vi "test Acyclic Loopback with SDI.vi"(8 "error in":errorcluster, 11 "TestCase in":refnum<class "Single Board Loopback.lvclass">) -> (0 "error out":errorcluster, 3 "TestCase out":refnum<class "Single Board Loopback.lvclass">)   [LabVIEW 2020, in "Single Board Loopback.lvclass"]
uses:
  Single Board Loopback.lvclass
  C:/Users/nitest/Desktop/Git 2020/niveristand-custom-device-testing-tools/VeriStandTestCase/VeriStandTestCase.lvclass
  <vilib>/numeric/Random Number (Range) U64.vi
  <vilib>/numeric/sub_Random U32.vi
  <vilib>/NI VeriStand/Execution/Workspace/NI VeriStand - Set Single Channel Value.vi
  <vilib>/addons/_JKI Toolkits/VI Tester/TestCase.llb/TestCase.lvclass
  <vilib>/NI VeriStand/Execution/Workspace/NI_VS Workspace ExecutionAPI.lvlib
  niveristand-custom-device-testing-tools/VeriStandTestUtilities/VeriStandTestUtilities.lvlib
  C:/Program Files (x86)/National Instruments/LabVIEW 2020/vi.lib/addons/_JKI Toolkits/VI Tester/TestCase.llb/TestCase.lvclass
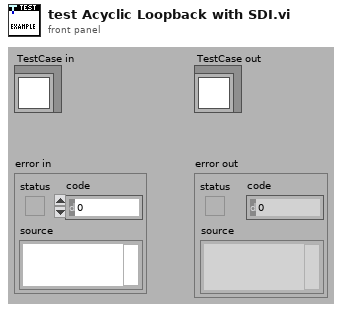
[diagram p1: front panel]
types:
  T1 = typedef "NI_VS Workspace ExecutionAPI.lvlib/WorkspaceAPI.ctl" = refnum<k24>
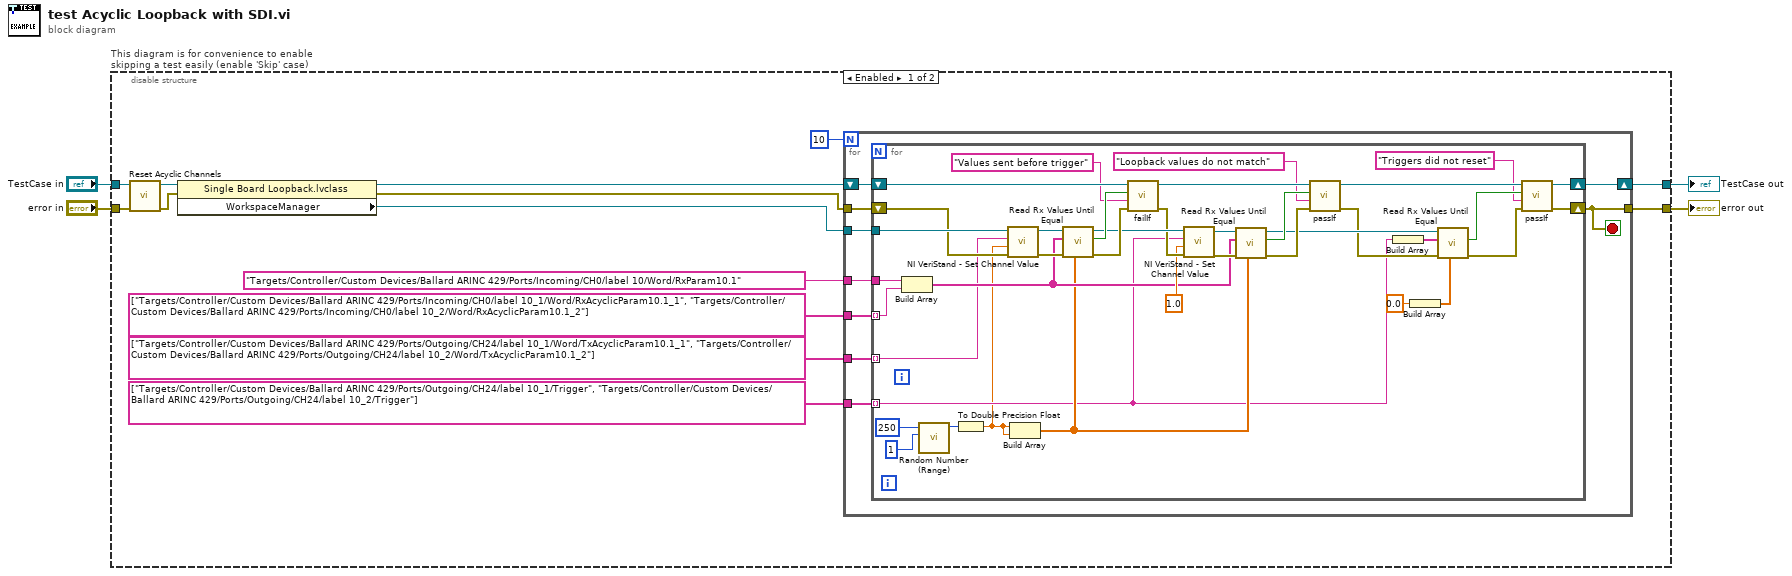
[diagram p0: block diagram]
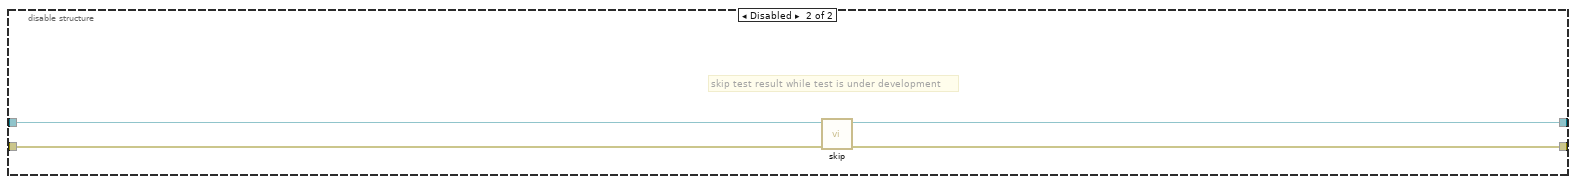
[diagram p2: hidden frame]
diagram:
  n1 = disable-structure "This diagram is for convenience to enable skipping a test easily (enable 'Skip' case)" shown="Enabled" {
    disable-tunnel: "TestCase in" -> [w9 w69]
    disable-tunnel: [w14 w67] -> w1
    disable-tunnel: [w13 w68] -> w3
    disable-tunnel: "error in" -> [w8 w66]
    frame Enabled {
      n2 = call "Reset Acyclic Channels.vi"("error in (no error)"=w8, "reference in"=w9) -> ("error out"=w6:errorcluster, "reference out"=w7:refnum<class "Single Board Loopback.lvclass">)  [unwired: 8 in]
      n3 = property class="Single Board Loopback.lvclass"(reference=w7, error in=w6) -> (reference out=w16:refnum<class "Single Board Loopback.lvclass">, error out=w17:errorcluster, "WorkspaceManager"=w18:T1)
      n4 = for {
        N: 10 -> [_]
        tunnel: w18 -> [w27]
        shift-right: [w23] -> w14
        shift-left: w16 -> [w26]
        tunnel: "Targets/Controller/Custom Devices/Ballard ARINC 429/Ports/Incoming/CH0/label 10/Word/RxParam10.1" -> [w22]
        tunnel: string[] ["Targets/Controller/Custom Devices/Ballard ARINC 429/Ports/Outgoing/CH24/label 10_1/Word/TxAcyclicParam10.1_1", "Targets/Controller/Custom Devices/Ballard ARINC 429/Ports/Outgoing/CH24/label 10_2/Word/TxAcyclicParam10.1_2"] -> [w21]
        tunnel: string[] ["Targets/Controller/Custom Devices/Ballard ARINC 429/Ports/Outgoing/CH24/label 10_1/Trigger", "Targets/Controller/Custom Devices/Ballard ARINC 429/Ports/Outgoing/CH24/label 10_2/Trigger"] -> [w20]
        tunnel: w17 -> [w25]
        tunnel: [w24] -> w13
        tunnel: string[] ["Targets/Controller/Custom Devices/Ballard ARINC 429/Ports/Incoming/CH0/label 10_1/Word/RxAcyclicParam10.1_1", "Targets/Controller/Custom Devices/Ballard ARINC 429/Ports/Incoming/CH0/label 10_2/Word/RxAcyclicParam10.1_2"] -> [w19]
        stop <- w24 stop-if-true
        n5 = for {
          tunnel: w27 -> [w64]
          tunnel: w22 -> [w40]
          shift-right: [w49] -> w23
          shift-left: w26 -> [w60]
          shift-right: [w30] -> w24
          shift-left: w25 -> [w58]
          tunnel: w21 -> [w35] mode=indexing
          tunnel: w20 -> [w34] mode=indexing
          tunnel: w19 -> [w29] mode=indexing
          n6 = Build Array(w40, w29) -> (w37:string[])
          n7 = call-poly <vilib>:"Random Number (Range).vi"("lower bound (0)"=u64 1 ("upper bound (100)"), "upper bound (100)"=u64 250) -> ("number"=w41:u64)  [unwired: 9 in]
          n8 = To Double Precision Float(number=w41) -> (double precision float=w28:dbl)
          n9 = call-poly <vilib>:"NI VeriStand - Set Channel Value.vi"("error in (no error)"=w58, "Value"=w28, "Channel"=w35, "WorkspaceManager in"=w64) -> ("error out"=w61:errorcluster, "WorkspaceManager out"=w63:T1)  [unwired: 6 in]
          n10 = Build Array(w28, w28) -> (w36:dbl[])
          n11 = call "Read Rx Values Until Equal.vi"("expected values"=w36, "error in"=w61, "Rx aliases"=w37, "workspace manager in"=w63) -> ("error out"=w62:errorcluster, "values equal expected"=w59:bool, "workspace manager out"=w57:T1)  [unwired: 5 in]
          n12 = call-dynamic "failIf.vi"("error in (no error)"=w62, "message (\"\")"="Values sent before trigger" ("message (\"\")"), "fail"=w59, "TestCase in"=w60) -> ("error out"=w56:errorcluster, "TestCase out"=w51:refnum<class "Single Board Loopback.lvclass">)  [unwired: 6 in]
          n13 = call-poly <vilib>:"NI VeriStand - Set Channel Value.vi"("error in (no error)"=w56, "Value"=1.0, "Channel"=w34, "WorkspaceManager in"=w57) -> ("error out"=w54:errorcluster, "WorkspaceManager out"=w55:T1)  [unwired: 6 in]
          n14 = call "Read Rx Values Until Equal.vi"("expected values"=w36, "error in"=w54, "Rx aliases"=w37, "workspace manager in"=w55) -> ("error out"=w52:errorcluster, "values equal expected"=w53:bool, "workspace manager out"=w47:T1)  [unwired: 5 in]
          n15 = call-dynamic "passIf.vi"("error in (no error)"=w52, "message (\"\")"="Loopback values do not match" ("message (\"\")"), "pass"=w53, "TestCase in"=w51) -> ("error out"=w46:errorcluster, "TestCase out"=w50:refnum<class "Single Board Loopback.lvclass">)  [unwired: 6 in]
          n16 = Build Array(w34) -> (w33:string[])
          n17 = Build Array(0.0) -> (w31:dbl[])
          n18 = call "Read Rx Values Until Equal.vi"("expected values"=w31, "error in"=w46, "Rx aliases"=w33, "workspace manager in"=w47) -> ("error out"=w45:errorcluster, "values equal expected"=w48:bool)  [unwired: 5 in, 1 out]
          n19 = call-dynamic "passIf.vi"("error in (no error)"=w45, "message (\"\")"="Triggers did not reset" ("message (\"\")"), "pass"=w48, "TestCase in"=w50) -> ("error out"=w30:errorcluster, "TestCase out"=w49:refnum<class "Single Board Loopback.lvclass">)  [unwired: 6 in]
        }
      }
    }
    frame Disabled {
      # "skip test result while test is under development"
      n20 = call <vilib>:"skip.vi"("error in (no error)"=w66, "TestCase in"=w69) -> ("error out"=w68:errorcluster, "TestCase out"=w67:refnum<class "Single Board Loopback.lvclass">)  [unwired: 8 in]
    }
  }
  "error out" <- w3
  "TestCase out" <- w1
